vi "Parallax PING Read Distance(0).vi"(8 "error in (no error)":errorcluster, 9 "stop":bool, 10 "Temperature (deg C)":dbl=25.0, 11 "myRIO DIO Channel":tag="C/DIO1") -> (0 "error out":errorcluster, 3 "Distance (cm)":dbl)   [LabVIEW 2017]
doc: "Reads the distance in meters from the Parallax PING sensor located on the given pin.\n\nReturns -1 if the distance could not be read."
uses:
  <vilib>/myRIO/Instrument Drivers/Onboard IO/DIO/typedefs/DIO Reference.ctl
  <vilib>/myRIO/Common/Instrument Driver Framework/Utilities/typedefs/myRIO Generic Hardware Reference.ctl
  <vilib>/myRIO/Common/Instrument Driver Framework/Utilities/typedefs/Hardware Version Enum.ctl
  <vilib>/myRIO/Common/Instrument Driver Framework/Utilities/typedefs/myRIO v1.0 Reference.ctl
  <vilib>/myRIO/Common/Instrument Driver Framework/Utilities/typedefs/Generic FPGA Reference.ctl
  <vilib>/myRIO/Common/Instrument Driver Framework/myRIO v1.0/DIO/typedefs/DIO Channels List.ctl
  <vilib>/myRIO/Common/Instrument Driver Framework/myRIO v1.0/DIO/typedefs/DIO Channels Enum.ctl
  <vilib>/myRIO/Common/Instrument Driver Framework/myRIO v1.0/DIO/vis/myRIO v1.0 Close DIO.vi
  <vilib>/myRIO/Common/Instrument Driver Framework/myRIO v1.0/DIO/vis/myRIO v1.0 Unreserve DIO.vi
  <vilib>/myRIO/Common/Instrument Driver Framework/myRIO v1.0/DIO/vis/myRIO v1.0 Build MUX Configuration DIO.vi
  <vilib>/myRIO/Common/Instrument Driver Framework/myRIO v1.0/Resource Manager/vis/myRIO v1.0 Unreserve Channel List.vi
  <vilib>/myRIO/Common/Instrument Driver Framework/myRIO v1.0/Resource Manager/vis/myRIO v1.0 Create Configuration List.vi
  <vilib>/myRIO/Common/Instrument Driver Framework/myRIO v1.0/Resource Manager/vis/myRIO v1.0 Unreserve Channel.vi
  <vilib>/myRIO/Common/Instrument Driver Framework/myRIO v1.0/Resource Manager/vis/myRIO v1.0 Build Mutex Name.vi
  <vilib>/Utility/error.llb/Error Cluster From Error Code.vi
  <vilib>/myRIO/Common/Instrument Driver Framework/myRIO v1.0/myRIO v1.0 Close.vi
  <vilib>/myRIO/Common/Instrument Driver Framework/Utilities/vis/IO Manager.vi
  <vilib>/myRIO/Common/Instrument Driver Framework/Utilities/vis/Configuration Manager.vi
  <vilib>/myRIO/Common/Instrument Driver Framework/myRIO v1.0/Resource Manager/vis/myRIO v1.0 Configure IO.vi
  <vilib>/myRIO/Common/Instrument Driver Framework/myRIO v1.0/DIO/vis/myRIO v1.0 Shutdown DIO.vi
  <vilib>/myRIO/Common/Instrument Driver Framework/myRIO v1.0/DIO/vis/myRIO v1.0 Read DIO.vi
  <vilib>/myRIO/Common/Instrument Driver Framework/myRIO v1.0/DIO/vis/myRIO v1.0 Write DIO.vi
  <vilib>/myRIO/Instrument Drivers/Onboard IO/DIO/DIO.lvlib
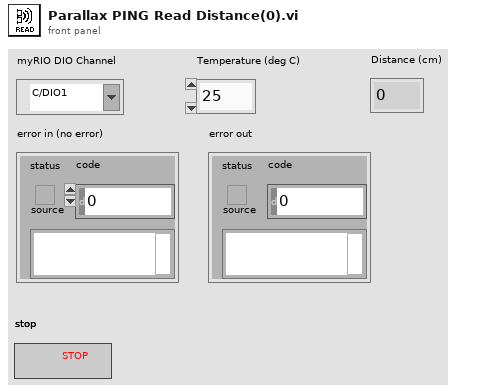
[diagram p1: front panel]
types:
  T1 = enum16{"Initialize", "Trigger pulse", "Wait for rising edge", "Wait for falling edge", "Calculate distance", "Stop"}
  T2 = typedef "DIO.lvlib/DIO Reference.ctl" = cluster{"myRIO Reference":T3, "DIO Channels List":T7}
  T3 = typedef "myRIO Generic Hardware Reference.ctl" = cluster{"myRIO Model":T4, "myRIO Hardware Reference":T5}
  T4 = typedef "Hardware Version Enum.ctl" = enum16{"Unknown", "myRIO-1900", "myRIO-1950", "roboRIO", "NI ELVIS RIO CM"}
  T5 = typedef "myRIO v1.0 Reference.ctl" = cluster{"Generic FPGA Reference":T6, "Allow multiple opens":bool}
  T6 = typedef "Generic FPGA Reference.ctl" = refnum<k20>
  T7 = typedef "DIO Channels List.ctl" = T8[]
  T8 = typedef "DIO Channels Enum.ctl" = enum16{"Not Connected", "C/DIO0", "C/DIO1", "C/DIO2", "C/DIO3", "C/DIO4", "C/DIO5", "C/DIO6", "C/DIO7", "A/DIO0", "A/DIO1", "A/DIO2", "A/DIO3", "A/DIO4", "A/DIO5", "A/DIO6", "A/DIO7", "A/DIO8", "A/DIO9", "A/DIO10", "A/DIO11", "A/DIO12", "A/DIO13", "A/DIO14", "A/DIO15", "B/DIO0", "B/DIO1", "B/DIO2", "B/DIO3", "B/DIO4", "B/DIO5", "B/DIO6", "B/DIO7", "B/DIO8", "B/DIO9", "B/DIO10", "B/DIO11", "B/DIO12", "B/DIO13", "B/DIO14", "B/DIO15", "LED0", "LED1", "LED2", "LED3", "Button0", "DIO/DIO0", "DIO/DIO1", "DIO/DIO2", "DIO/DIO3", "DIO/DIO4", "DIO/DIO5", "DIO/DIO6", "DIO/DIO7", "DIO/DIO8", "DIO/DIO9", "SPI/CS0", "SPI/CS1", "SPI/CS2", "SPI/CS3", "LED RADIO (Green)", "LED RADIO (Red)", "LED COMM (Green)", "LED COMM (Red)", "LED MODE (Green)", "LED MODE (Red)"}
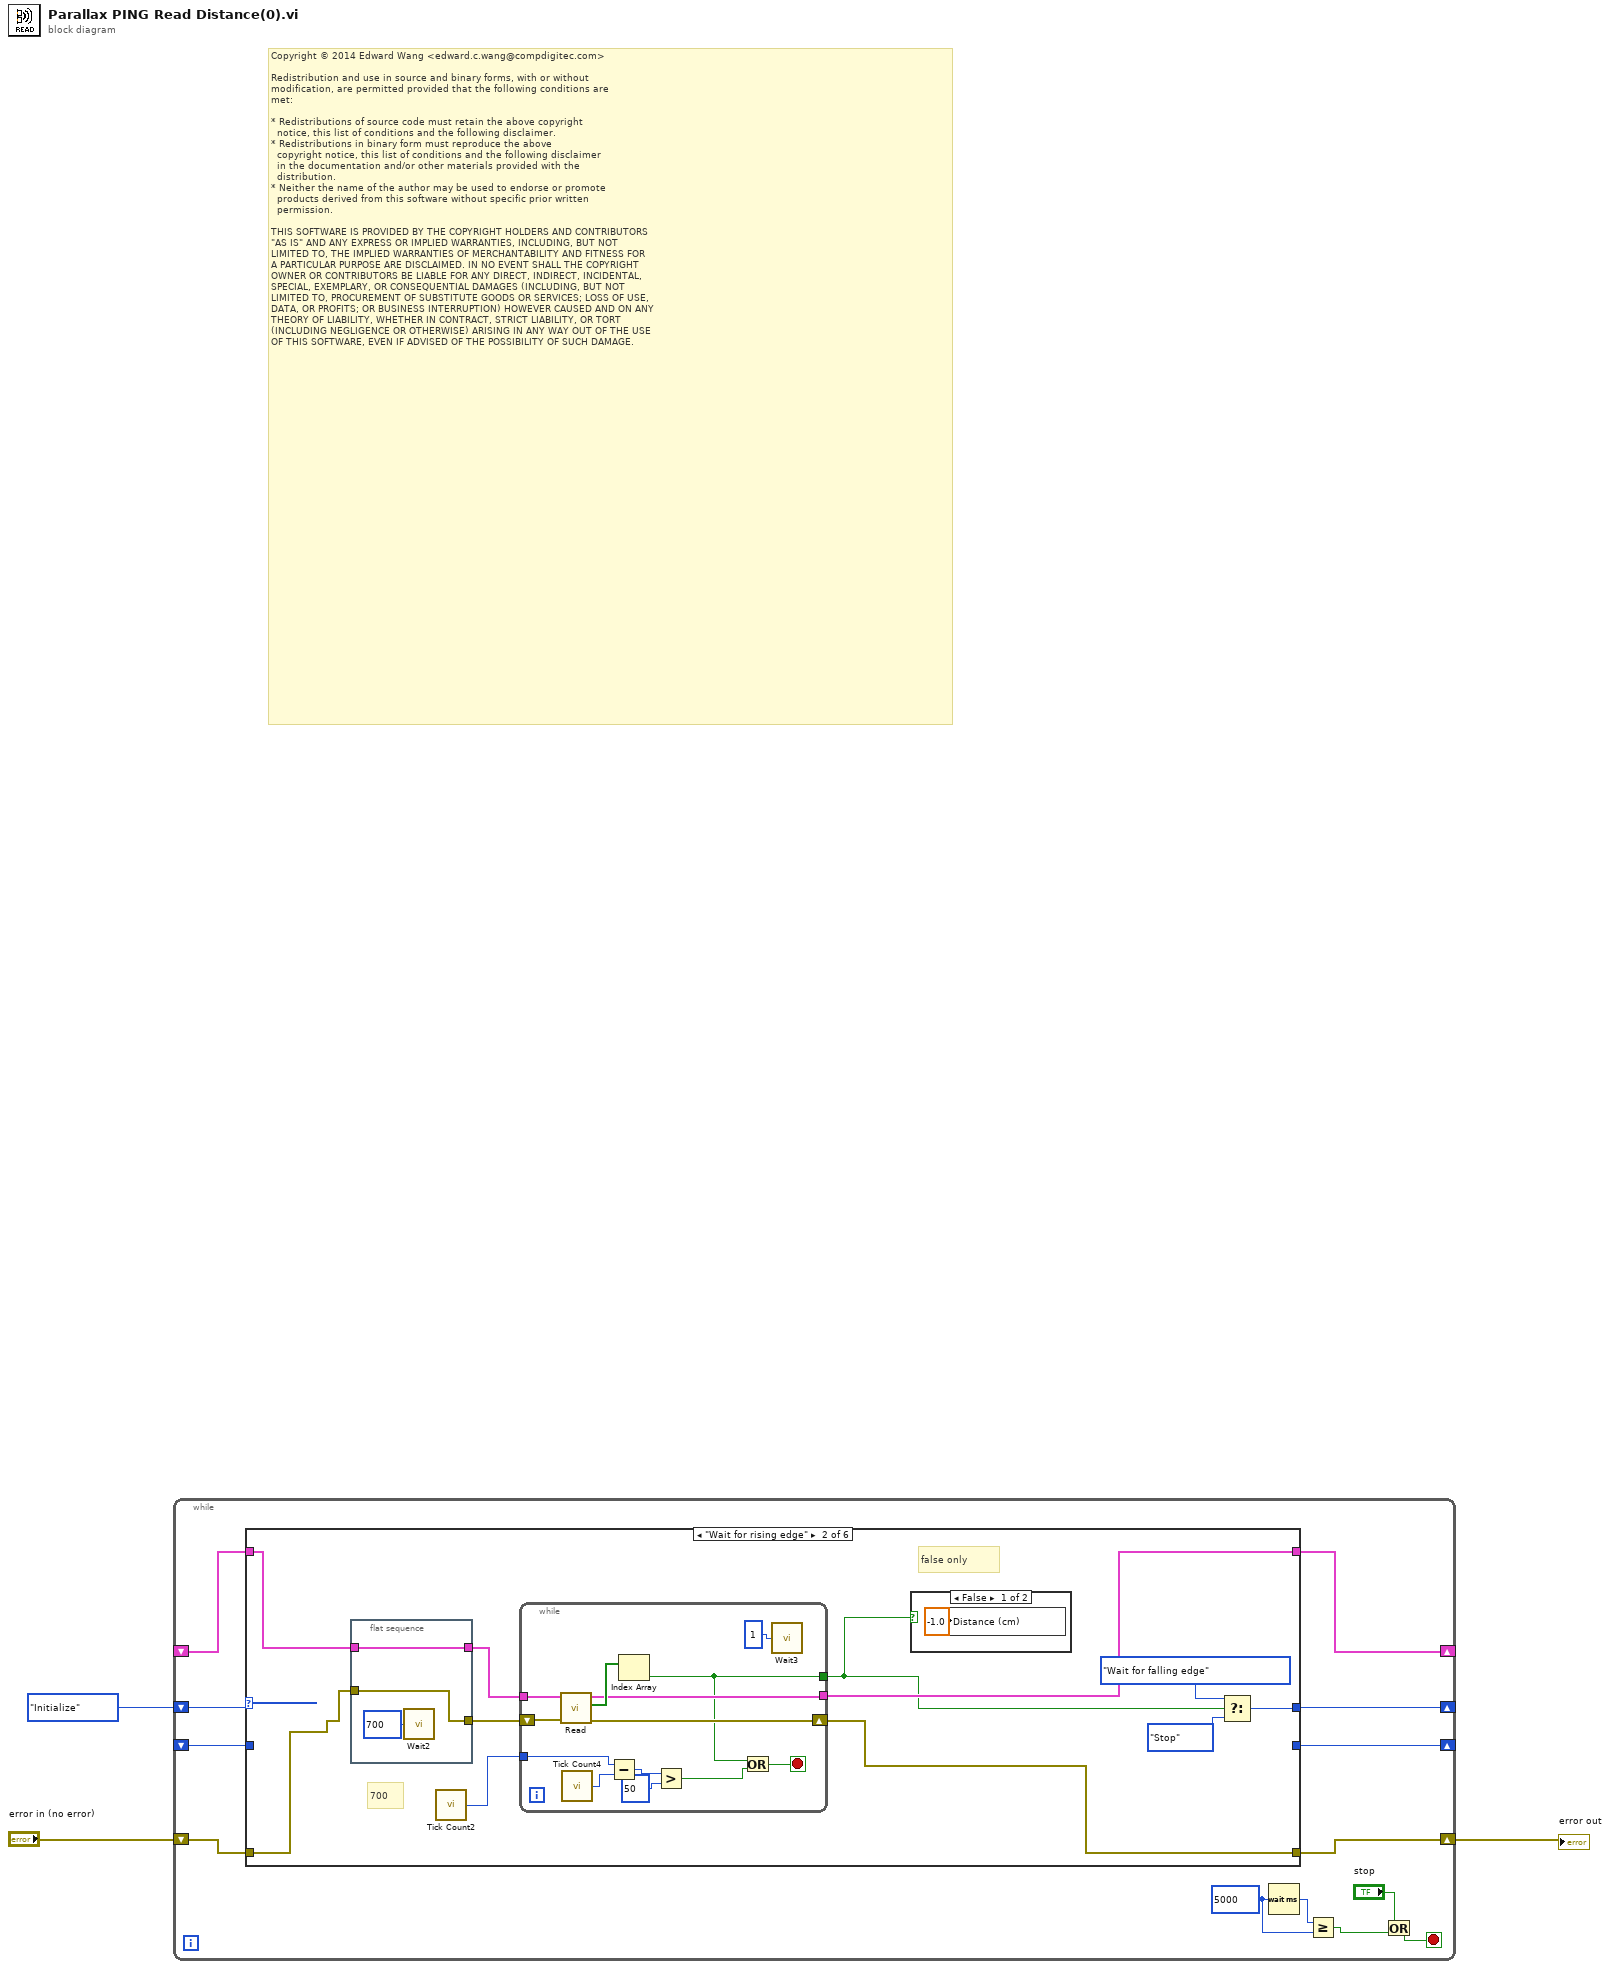
[diagram p0: block diagram]
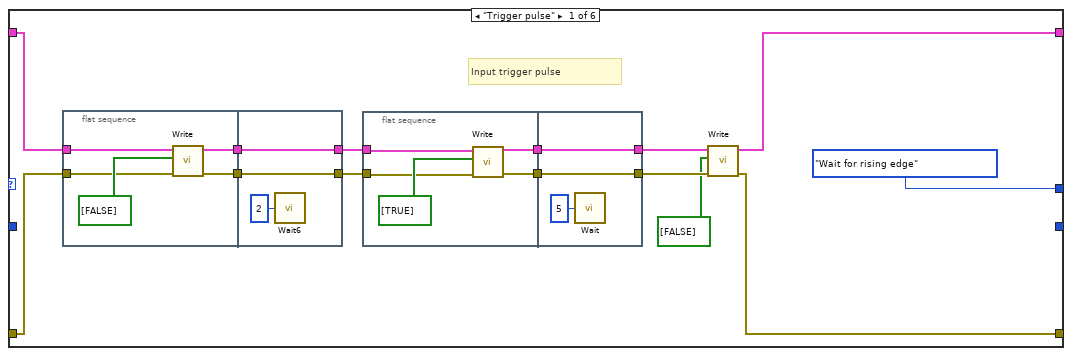
[diagram p2: hidden frame]
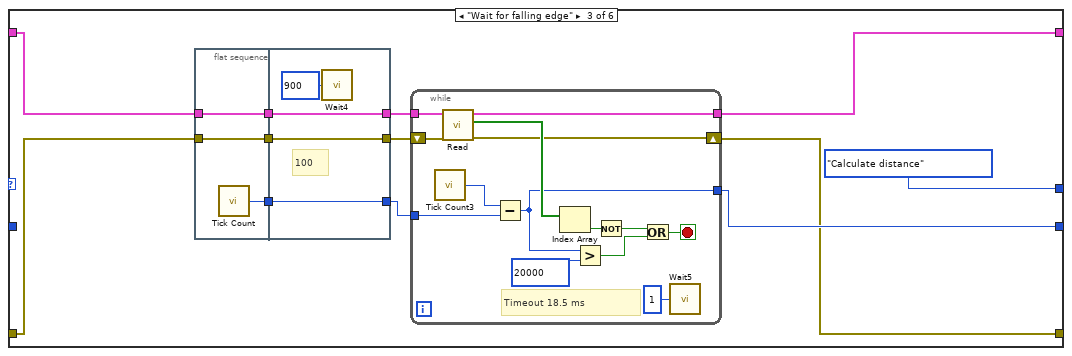
[diagram p4: hidden frame]
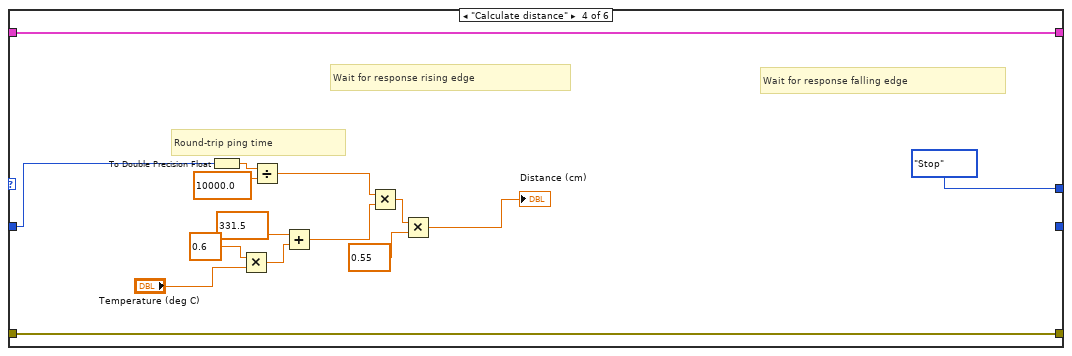
[diagram p5: hidden frame]
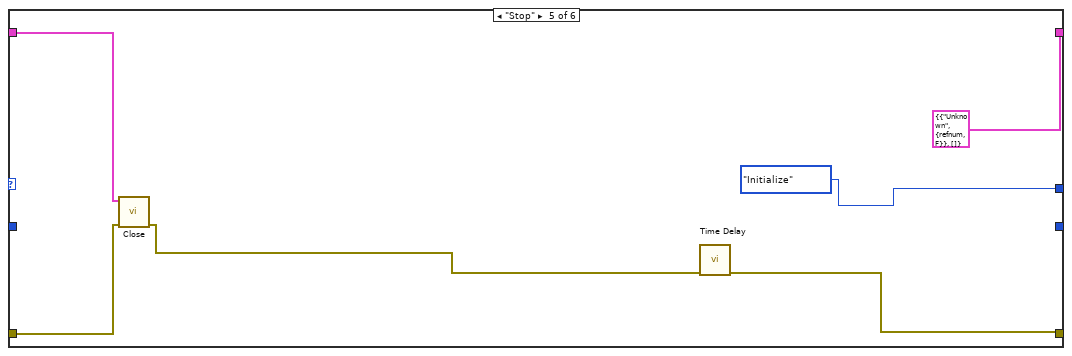
[diagram p6: hidden frame]
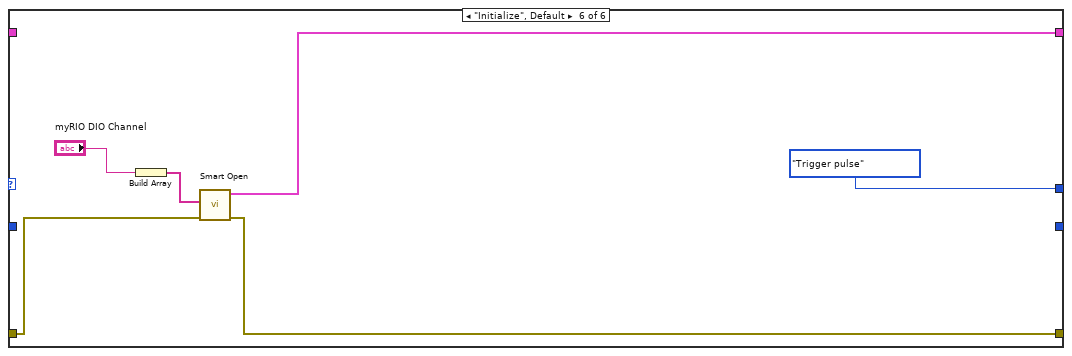
[diagram p7: hidden frame]
diagram:
  # "Copyright © 2014 Edward Wang <edward.c.wang@compdigitec.com>\n\nRedistribution and use in source and binary forms, with or without\nmodification, are permitted provided that the following conditions are\nmet:\n\n* Redistributions of source code must retain the above copyright\n  notice, this list of conditions and the following disclaimer.\n* Redistributions in binary form must reproduce the above\n  copyright notice, this list of conditions and the following disclaimer\n  in the documentation and/or other materials provided with the\n  distribution.\n* Neither the name of the author may be used to endorse or promote\n  products derived from this software without specific prior written\n  permission.\n\nTHIS SOFTWARE IS PROVIDED BY THE COPYRIGHT HOLDERS AND CONTRIBUTORS\n\"AS IS\" AND ANY EXPRESS OR IMPLIED WARRANTIES, INCLUDING, BUT NOT\nLIMITED TO, THE IMPLIED WARRANTIES OF MERCHANTABILITY AND FITNESS FOR\nA PARTICULAR PURPOSE ARE DISCLAIMED. IN NO EVENT SHALL THE COPYRIGHT\nOWNER OR CONTRIBUTORS BE LIABLE FOR ANY DIRECT, INDIRECT, INCIDENTAL,\nSPECIAL, EXEMPLARY, OR CONSEQUENTIAL DAMAGES (INCLUDING, BUT NOT\nLIMITED TO, PROCUREMENT OF SUBSTITUTE GOODS OR SERVICES; LOSS OF USE,\nDATA, OR PROFITS; OR BUSINESS INTERRUPTION) HOWEVER CAUSED AND ON ANY\nTHEORY OF LIABILITY, WHETHER IN CONTRACT, STRICT LIABILITY, OR TORT\n(INCLUDING NEGLIGENCE OR OTHERWISE) ARISING IN ANY WAY OUT OF THE USE\nOF THIS SOFTWARE, EVEN IF ADVISED OF THE POSSIBILITY OF SUCH DAMAGE."
  n1 = while {
    shift-right: [w10] -> _
    shift-left: T1."Initialize" -> [w16]
    shift-right: [w12] -> w1
    shift-left: "error in (no error)" -> [w15]
    shift-right: [w14] -> _
    shift-left: _ -> [w13]
    shift-right: [w8] -> _
    shift-left: _ -> [w11]
    stop <- w5 stop-if-true
    w6 = u32 5000 ("milliseconds to wait")
    n2 = case shown="\"Wait for rising edge\"" w16 {
      tunnel: [T1."Wait for rising edge" w48 T1."Calculate distance" ("y") T1."Stop" ("y") T1."Initialize" ("y") T1."Trigger pulse"] -> w10
      tunnel: w15 -> [w21 w53 w79 w110 w128 w132]
      tunnel: [w19 w57 w78 w122 T2 {"myRIO Reference"={"myRIO Model"=enum."Unknown", "myRIO Hardware Reference"={"Generic FPGA Reference"=refnum, "Allow multiple opens"=FALSE}}, "DIO Channels List"=[]} ("DIO Ref Out") w131] -> w14
      tunnel: w13 -> [w20 w52 w80 w122 w127 _]
      tunnel: [w18 w56 w75 w110 w123 w130] -> w12
      tunnel: [_ _ w77 _ _ _] -> w8
      tunnel: w11 -> [_ _ _ w109 _ _]
      frame "Trigger pulse" {
        # "Input trigger pulse"
        n3 = flat-sequence {
          tunnel: [w34] -> w28
          tunnel: [w33] -> w27
          tunnel: w21 -> [w32]
          tunnel: w20 -> [w31]
          tunnel: [w37] -> w25
          tunnel: [w36] -> w26
          tunnel: w28 -> [w37]
          tunnel: w27 -> [w36]
          frame #0 {
            n4 = call <vilib>:"Write.vi"("error in (no error)"=w32, "Values"=bool[] [FALSE], "DIO Ref In"=w31) -> ("error out"=w33:errorcluster, "DIO Ref Out"=w34:T2)  [unwired: 6 in]
          }
          frame #1 {
            n5 = call "Wait6"("Count(uSec)"=u32 2) -> ()  [unwired: 1 out]
          }
        }
        n6 = flat-sequence {
          tunnel: [w42] -> w30
          tunnel: [w41] -> w29
          tunnel: w26 -> [w40]
          tunnel: w25 -> [w39]
          tunnel: [w45] -> w22
          tunnel: [w44] -> w24
          tunnel: w30 -> [w45]
          tunnel: w29 -> [w44]
          frame #0 {
            n7 = call <vilib>:"Write.vi"("error in (no error)"=w40, "Values"=bool[] [TRUE], "DIO Ref In"=w39) -> ("error out"=w41:errorcluster, "DIO Ref Out"=w42:T2)  [unwired: 6 in]
          }
          frame #1 {
            n8 = call "Wait"("Count(uSec)"=u32 5) -> ()  [unwired: 1 out]
          }
        }
        n9 = call <vilib>:"Write.vi"("error in (no error)"=w24, "Values"=bool[] [FALSE], "DIO Ref In"=w22) -> ("error out"=w18:errorcluster, "DIO Ref Out"=w19:T2)  [unwired: 6 in]
      }
      frame "Wait for rising edge" {
        # "700"
        # "false only"
        n10 = flat-sequence {
          tunnel: [w60] -> w54
          tunnel: w53 -> [w60]
          tunnel: w52 -> [w59]
          tunnel: [w59] -> w51
          frame #0 {
            n11 = call "Wait2"("Count(uSec)"=u32 700) -> ()  [unwired: 1 out]
          }
        }
        n12 = call "Tick Count2"() -> ("Tick Count(uSec)"=w55:u32)
        n13 = while {
          tunnel: [w72] -> w57
          shift-right: [w70] -> w56
          shift-left: w54 -> [w71]
          tunnel: w55 -> [w67]
          tunnel: w51 -> [w69]
          tunnel: [w62] -> w47
          stop <- w64 stop-if-true
          n14 = call <vilib>:"Read.vi"("error in (no error)"=w71, "DIO Ref In"=w69) -> ("error out"=w70:errorcluster, "Values"=w73:bool[], "DIO Ref Out"=w72:T2)  [unwired: 7 in]
          n15 = call "Tick Count4"() -> ("Tick Count(uSec)"=w68:u32)
          n16 = Subtract(x=w67, y=w68) -> (x-y=w66:u32)
          n17 = Index Array(array=w73) -> (element=w62:bool)  [unwired: 1 in]
          n18 = Greater?(x=w66, y=u32 50) -> (0:w63:bool)
          n19 = Or(x=w62, y=w63) -> (x .or. y?=w64:bool)
          n20 = call "Wait3"("Count(uSec)"=u32 1) -> ()  [unwired: 1 out]
        }
        n21 = case shown="False" w47 {
          frame False {
            n22 = local write "Distance (cm)"(-1.0 ("Distance (m)")) -> ()
          }
          frame True {
          }
        }
        n23 = Select(t=T1."Wait for falling edge", s=w47, f=T1."Stop" ("y")) -> (s? t:f=w48:T1)
      }
      frame "Wait for falling edge" {
        n24 = flat-sequence {
          tunnel: w80 -> [w103]
          tunnel: [w103] -> w86
          tunnel: [w102] -> w85
          tunnel: [w101] -> w84
          tunnel: w79 -> [w101]
          tunnel: [w106] -> w82
          tunnel: [w107] -> w83
          tunnel: w86 -> [w107]
          tunnel: w85 -> [w106]
          tunnel: w84 -> [w104]
          tunnel: [w104] -> w81
          frame #0 {
            n25 = call "Tick Count"() -> ("Tick Count(uSec)"=w102:u32)
          }
          frame #1 {
            # "100"
            n26 = call "Wait4"("Count(uSec)"=u32 900) -> ()  [unwired: 1 out]
          }
        }
        n27 = while {
          tunnel: w83 -> [w99]
          tunnel: w82 -> [w96]
          shift-right: [w90] -> w75
          shift-left: w81 -> [w91]
          tunnel: [w88] -> w78
          tunnel: [w87] -> w77
          stop <- w95 stop-if-true
          # "Timeout 18.5 ms"
          n28 = call "Tick Count3"() -> ("Tick Count(uSec)"=w89:u32)
          n29 = call <vilib>:"Read.vi"("error in (no error)"=w91, "DIO Ref In"=w99) -> ("error out"=w90:errorcluster, "Values"=w98:bool[], "DIO Ref Out"=w88:T2)  [unwired: 7 in]
          n30 = Subtract(x=w89, y=w96) -> (x-y=w87:u32)
          n31 = Index Array(array=w98) -> (element=w97:bool)  [unwired: 1 in]
          n32 = Greater?(x=w87, y=u32 20000) -> (0:w93:bool)
          n33 = Not(x=w97) -> (.not. x?=w94:bool)
          n34 = Or(x=w94, y=w93) -> (x .or. y?=w95:bool)
          n35 = call "Wait5"("Count(uSec)"=u32 1) -> ()  [unwired: 1 out]
        }
      }
      frame "Calculate distance" {
        # "Wait for response falling edge"
        # "Wait for response rising edge"
        # "Round-trip ping time"
        n36 = To Double Precision Float(number=w109) -> (double precision float=w117:dbl)
        n37 = Multiply(x=0.6, y="Temperature (deg C)") -> (x*y=w115:dbl)
        n38 = Divide(x=w117, y=10000.0) -> (x/y=w119:dbl)
        n39 = Add(x=331.5, y=w115) -> (x+y=w120:dbl)
        n40 = Multiply(x=w119, y=w120) -> (x*y=w112:dbl)
        n41 = Multiply(x=w112, y=0.55) -> (x*y=→"Distance (cm)":dbl)
      }
      frame "Stop" {
        n42 = call <vilib>:"Close.vi"("error in (no error)"=w128, "DIO Ref In"=w127) -> ("error out"=w124:errorcluster)  [unwired: 9 in]
        n43 = call "Time Delay"("error in (no error)"=w124) -> ("error out"=w123:errorcluster)  [unwired: 10 in]
      }
      frame "Initialize", Default {
        n44 = Build Array("myRIO DIO Channel") -> (w134:tag[])
        n45 = call <vilib>:"Smart Open.vi"("error in (no error)"=w132, "Channel Names"=w134) -> ("error out"=w130:errorcluster, "DIO Ref Out"=w131:T2)  [unwired: 8 in]
      }
    }
    n46 = Wait (ms)(milliseconds to wait=w6) -> (millisecond timer value=w7:u32)
    n47 = Greater Or Equal?(x=w7, y=w6) -> (x >= y?=w4:bool)
    n48 = Or(x="stop", y=w4) -> (x .or. y?=w5:bool)
  }
  "error out" <- w1
